vi "FormatPayload.vi"(4 "mask":bool=TRUE, 5 "final":bool=TRUE, 6 "mask value":u32 format="%.0x", 7 "opcode":T1=enum."Close", 10 "payload":string) -> (2 "packet":string)   [LabVIEW 2014, in "Raspberry Pi Compatible Compiler for LabVIEW.lvlib" / "Websocket.lvlib"]
uses:
  Websocket.lvlib
  WebsocketFrameTypes_TD.ctl
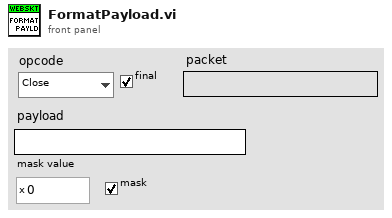
[diagram p1: front panel]
types:
  T1 = typedef "Raspberry Pi Compatible Compiler for LabVIEW.lvlib/Websocket.lvlib/WebsocketFrameTypes_TD.ctl" = enum8{"Continuation", "Text", "Binary", "Reserved 1", "Reserved 2", "Reserved 3", "Reserved 4", "Reserved 5", "Close", "Ping", "Pong", "Reserved 6", "Reserved 7", "Reserved 8", "Reserved 9", "Reserved 10"}
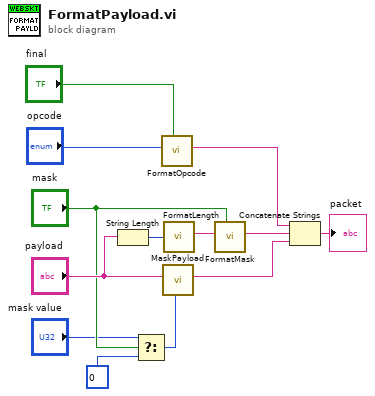
[diagram p0: block diagram]
diagram:
  n1 = String Length(string="payload") -> (length=w13:i32)
  n2 = Select(t="mask value", s="mask", f=u32 0) -> (s? t:f=w3:u32)
  n3 = call "FormatOpcode.vi"("final"="final", "opcode"="opcode") -> ("opcode"=w11:string)  [unwired: 7 in]
  n4 = call "MaskPayload.vi"("mask value"=w3, "payload"="payload") -> ("masked payload"=w10:string)  [unwired: 7 in]
  n5 = call "FormatLength.vi"("length"=w13) -> ("encoded length"=w9:string)  [unwired: 10 in]
  n6 = call "FormatMask.vi"("mask"="mask", "encoded length"=w9) -> ("encoded length with mask"=w8:string)  [unwired: 7 in]
  n7 = Concatenate Strings(w11, w8, w10) -> (→"packet":string)
